vi "CSM - Wait and Send Message for Reply.vi"(0 "State":string="API State", 1 "Current Module(\"\" to generate a ID)":string, 5 "Arguments (\"\")":string, 7 "Target Module":string="Target", 9 "Wait(5000ms)":i32=5000, 11 "Error In (no error)":errorcluster, 12 "Response Timeout(5000ms)":i32=5000) -> (6 "Response":string="DoA", 14 ">> Source CSM >>":string, 15 "error out":errorcluster)   [LabVIEW 2020, in "Communicable State Machine.lvlib"]
doc: "Send a message to CSM specified and wait for the reply with timeout.\n\n<b>Inputs:</b>\n - <b>Target Module</b>: Target CSM Module name.\n - <b>State</b>: Message to send\n - <b>Arguments (\"\")</b>: Argument of the message.\n - <b>Response Timeout(5000ms)</b>: Timeout for waiting the response.\n - <b>Error In (no error)</b>: Error cluster\n\n<b>Outputs:</b>\n - <b>Arguments</b>: Response returned.\n - <b>error out</b>: Error cluster"
uses:
  Communicable State Machine.lvlib
  Priority Queue.lvclass/Priority Queue.ctl
  CSM - Check If Module Exists.vi
  Build Error Cluster.vi
  CSMP-Sync Call.vi
  uuid.vi
  Trim Both Whitespace.vi
  _Obtain CSM Data Queue.vi
  Release Priority Queue.vi
  _CSMObj-Message Check.vi
  _CSMObj-Enqueue Cross-Module Message.vi
  _CSMOFGV Get.vi
  Obtain Priority Queue.vi
  Enqueue Element.vi
  CSM No Target Error.vi
  _CSMOFGV.vi
  CSM Not Allowed Message.vi
  CSM Target Error.vi
  CSM Unhandled State Error.vi
  CSM Target Timeout Error.vi
  Priority Queue.lvclass
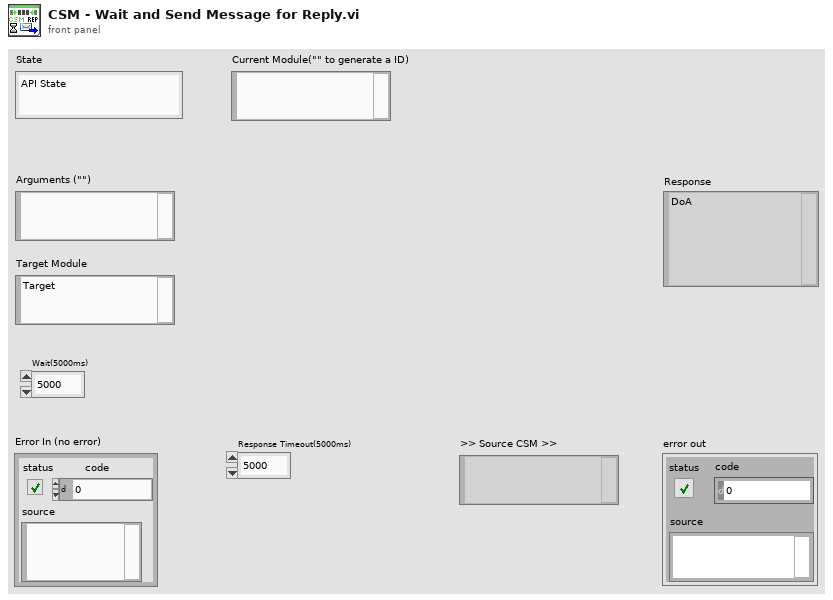
[diagram p1: front panel]
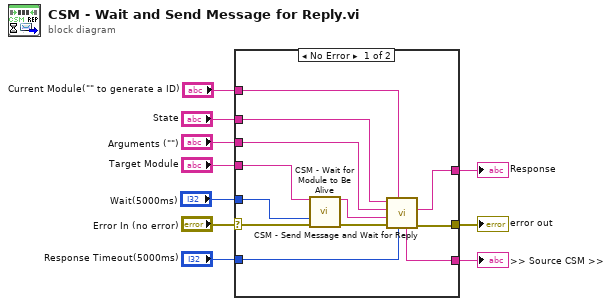
[diagram p0: block diagram]
diagram:
  n1 = case shown="No Error" "Error In (no error)" {
    selector: "Error In (no error)" -> [w22 w23]
    tunnel: "State" -> [w16 _]
    tunnel: "Response Timeout(5000ms)" -> [w11 _]
    tunnel: [w14 w23] -> w7
    tunnel: [w13 _] -> w6
    tunnel: "Target Module" -> [w21 _]
    tunnel: "Arguments (\"\")" -> [w17 _]
    tunnel: "Current Module(\"\" to generate a ID)" -> [w15 _]
    tunnel: [w12 _] -> w2
    tunnel: "Wait(5000ms)" -> [w20 _]
    frame No Error {
      n2 = call "CSM - Wait for Module to Be Alive.vi"("Target Module"=w21, "Wait(5000ms)"=w20, "error in (no error)"=w22) -> ("Target Module (dup)"=w18:string, "error out"=w19:errorcluster)  [unwired: 10 in, 1 out]
      n3 = call "CSM - Send Message and Wait for Reply.vi"("Response Timeout(5000ms)"=w11, "Current Module(\"\" to generate a ID)"=w15, "Error In (no error)"=w19, "Target Module"=w18, "Arguments (\"\")"=w17, "State"=w16) -> ("error out"=w14:errorcluster, "Response"=w13:string, ">> Source CSM >>"=w12:string)  [unwired: 3 in]
    }
    frame Error {
    }
  }
  "error out" <- w7
  "Response" <- w6
  ">> Source CSM >>" <- w2
